vi "TiePie.Lst.LstDevGetTypes.vi"(8 "error in (no error)":errorcluster, 10 "dwId":u32, 11 "dwIdKind":u32) -> (0 "error out":errorcluster)   [LabVIEW 2014, in "LVTiePie.lvlib"]
uses:
  LVTiePie.lvlib
  bin/libtiepie.dll
panel:
  out "deviceTypes":u32
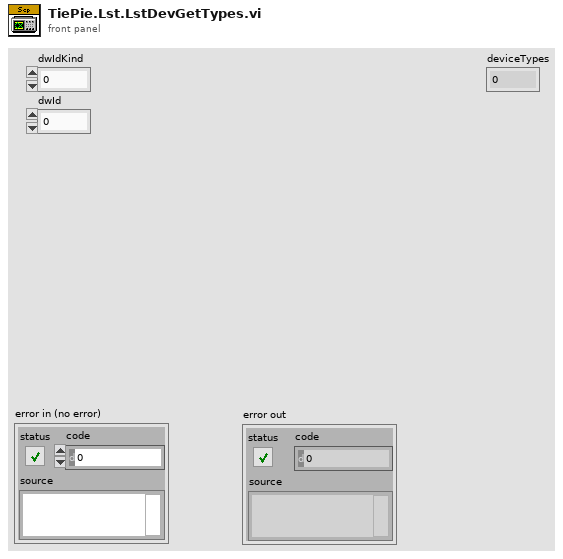
[diagram p1: front panel]
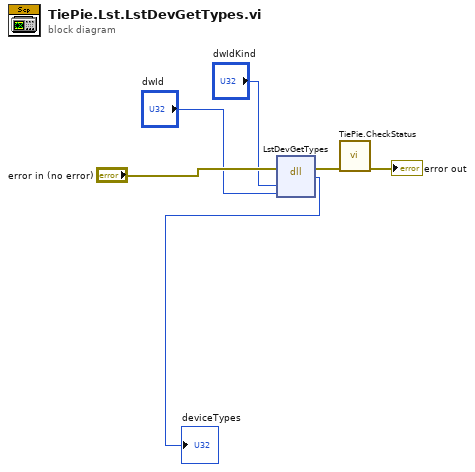
[diagram p0: block diagram]
diagram:
  n1 = dll-call lib="C:/Users/mbirski/Desktop/PAN/LabVEW/Tie Pie/bin/libtiepie.dll" fn="LstDevGetTypes"(error in="error in (no error)", "dwIdKind"="dwIdKind", "dwId"="dwId") -> (error out=w5:errorcluster, "deviceTypes"=→"deviceTypes":u32)  [unwired: 4 in, 1 out]
  n2 = call "TiePie.CheckStatus.vi"("error in (no error)"=w5) -> ("error out"=→"error out":errorcluster)  [unwired: 10 in]
